vi "NAN_REMOVE_1D.vi"(11 "Array 2":dbl[](array[numeric])=[1.0, 2.0, nan]) -> (3 "Array":dbl[](array[numeric]))   [LabVIEW 2019, in "Zen Analytics.lvlib" / "Zen Analytics.lvclass"]
uses:
  Zen Analytics.lvclass
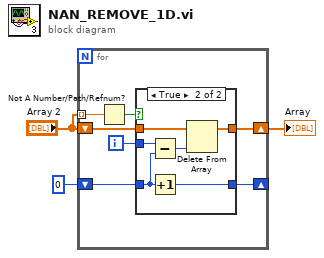
[diagram p0: block diagram]
diagram:
  n1 = for {
    tunnel: "Array 2" -> [w10] mode=indexing
    shift-right: [w7] -> _
    shift-left: 0 -> [w8]
    shift-right: [w4] -> w2
    shift-left: "Array 2" -> [w5]
    i -> [w6]
    n2 = Not A Number/Path/Refnum?(number/path/refnum=w10) -> (NaN/Path/Refnum?=w9:bool)
    n3 = case shown="True" w9 {
      tunnel: w5 -> [w11 w18]
      tunnel: w8 -> [w12 w13]
      tunnel: [w12 w16] -> w7
      tunnel: [w11 w17] -> w4
      tunnel: w6 -> [_ w14]
      frame False {
      }
      frame True {
        n4 = Subtract(x=w14, y=w13) -> (x-y=w15:i32)
        n5 = Increment(x=w13) -> (x+1=w16:i32)
        n6 = Delete From Array(array=w18, index=w15) -> (array with subset deleted=w17:dbl[])  [unwired: 1 in, 1 out]
      }
    }
  }
  "Array" <- w2
